vi "DecimalToBinaryArrayGraph.vi"() -> ()   [LabVIEW 2021]
panel:
  out "reversed array":i16[](array[numeric])
  out "Waveform Graph":i16[](graph)
  out "0, 1":i16[](array[numeric])
  out "Boolean array":bool[](array[boolean])
  in  "Number":u8
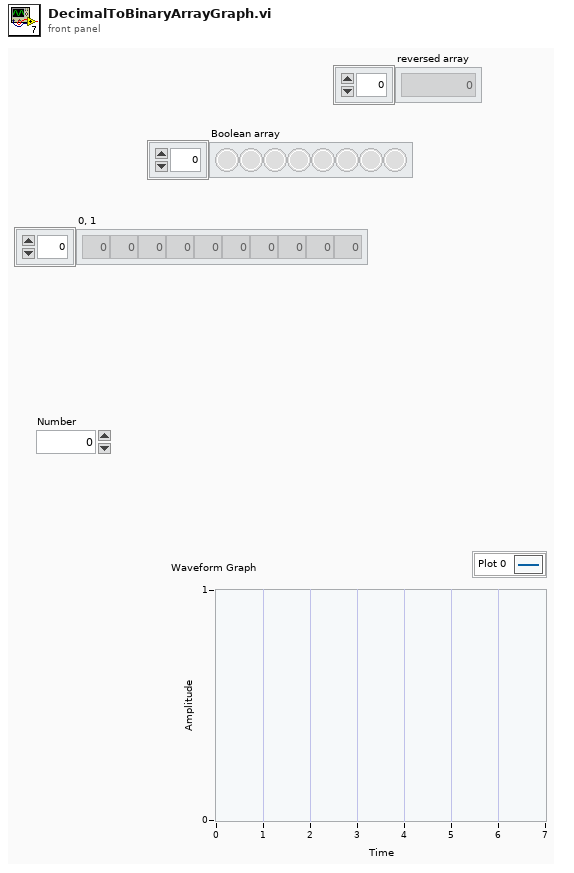
[diagram p1: front panel]
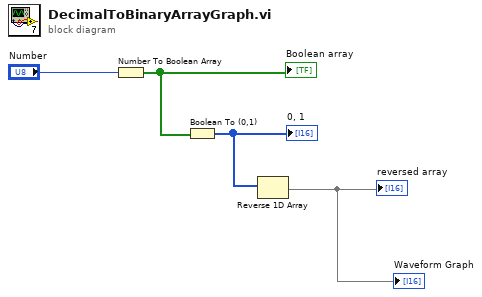
[diagram p0: block diagram]
diagram:
  n1 = Number To Boolean Array(number="Number") -> (Boolean array=w3:bool[])
  "Boolean array" <- w3
  n2 = Boolean To (0,1)(Boolean=w3) -> (0, 1=w2:i16[])
  "0, 1" <- w2
  n3 = Reverse 1D Array(array=w2) -> (reversed array=→"Waveform Graph" →"reversed array":i16[])
